vi "Post-Build Action.vi"(5 "Files Generated by Build":path[](array[path]), 6 "Top Level/Always Included VIs":path[](array[path]), 7 "Destination Path":path, 8 "error in (no error)":errorcluster, 9 "Target Name":string, 10 "Build Specification Name":string, 11 "Project Path":path) -> (0 "error out":errorcluster)   [LabVIEW 2019]
uses:
  <vilib>/Utility/sysdir.llb/System Directory Type.ctl
  <vilib>/Utility/config.llb/Write Key (String).vi
  <vilib>/Utility/config.llb/Write Key (I32).vi
  <vilib>/Utility/config.llb/NI_LVConfig.lvlib
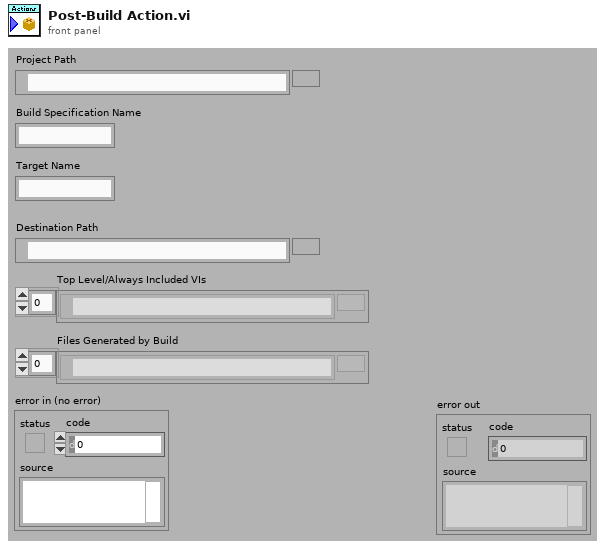
[diagram p1: front panel]
types:
  T1 = typedef "System Directory Type.ctl" = i32
  T2 = typedef "NI_LVConfig.lvlib/Config Data RefNum.ctl" = refnum<k1>
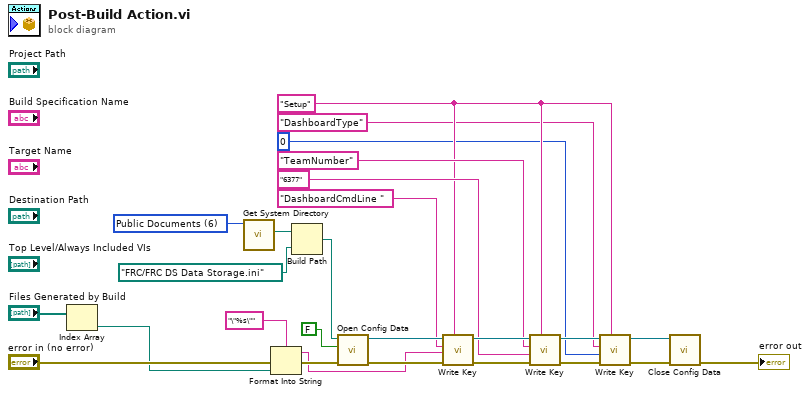
[diagram p0: block diagram]
diagram:
  w3 = "Setup" ("section")
  w26 = T1 6 items=["User Home"=0, "User Desktop"=1, "User Documents"=2, "User Application Data"=3, "User Preferences"=4, "User Temporary"=5, "Public Documents"=6, "Public Application Data"=7, "Public Preferences"=8, "Public Cache"=13, "System Core Libraries"=9, "System Installed Libraries"=10, "Application Files"=11, "Boot Volume Root"=12] ("system directory type")
  n1 = Index Array(array="Files Generated by Build") -> (element=w9:path)  [unwired: 1 in]
  n2 = call <vilib>:"Get System Directory.vi"("system directory type"=w26) -> ("system directory"=w25:path)  [unwired: 10 in]
  n3 = Format Into String(format string="\"%s\"", error in="error in (no error)", w9) -> (resulting string=w11:string, error out=w12:errorcluster)  [unwired: 1 in]
  n4 = Build Path(base path=w25, name or relative path=path "FRC/FRC DS Data Storage.ini") -> (appended path=w16:path)
  n5 = call <vilib>:"Open Config Data.vi"("error in (no error)"=w12, "create file if necessary (T)"=FALSE, "configuration file path"=w16) -> ("error out"=w22:errorcluster, "refnum"=w23:T2)  [unwired: 6 in, 1 out]
  n6 = call-poly <vilib>:"Write Key.vi"("section"=w3, "error in (no error)"=w22, "value"=w11, "key"="DashboardCmdLine ", "refnum"=w23) -> ("error out"=w20:errorcluster, "refnum out"=w21:T2)  [unwired: 4 in, 1 out]
  n7 = call-poly <vilib>:"Write Key.vi"("section"=w3, "error in (no error)"=w20, "value"="6377" ("key"), "key"="TeamNumber", "refnum"=w21) -> ("error out"=w19:errorcluster, "refnum out"=w5:T2)  [unwired: 4 in, 1 out]
  n8 = call-poly <vilib>:"Write Key.vi"("section"=w3, "error in (no error)"=w19, "value"=0, "key"="DashboardType" ("section"), "refnum"=w5) -> ("error out"=w6:errorcluster, "refnum out"=w4:T2)  [unwired: 4 in, 1 out]
  n9 = call <vilib>:"Close Config Data.vi"("error in (no error)"=w6, "refnum"=w4) -> ("error out"=→"error out":errorcluster)  [unwired: 8 in, 1 out]
